vi "лаба6.vi"() -> ()   [LabVIEW 2019]
panel:
  in  "stop":bool
  in  "Амплитуда":dbl(knob) scale=0.0..10.0
  out "Waveform Graph":dynamicdata(graph)
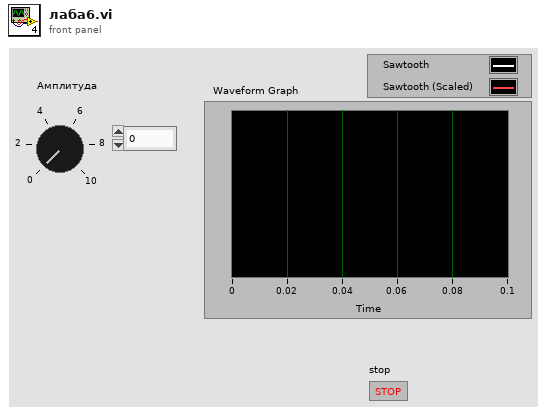
[diagram p1: front panel]
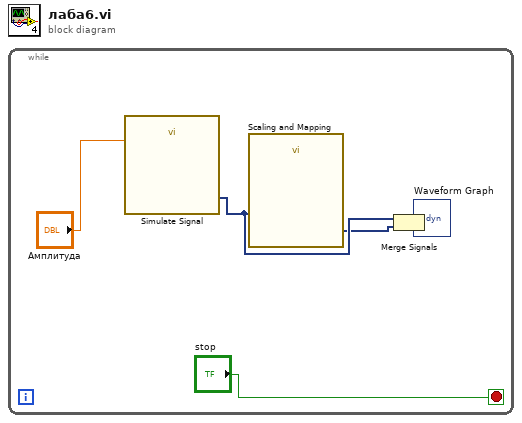
[diagram p0: block diagram]
diagram:
  n1 = while {
    stop <- "stop" stop-if-true
    n2 = call "Simulate Signal"("Amplitude"="Амплитуда") -> ("Sawtooth"=w4:dynamicdata)  [unwired: 13 in, 1 out]
    n3 = call "Scaling and Mapping"("Signals"=w4) -> ("Scaled Signals"=w2:dynamicdata)  [unwired: 9 in, 1 out]
    n4 = Merge Signals(w4, w2) -> (→"Waveform Graph":dynamicdata)
  }
